vi "四段比较器（TimeStamp[]）.vi"(1 "输入时间标识":timestamp[](array[timestamp]), 2 "低":timestamp, 3 "中":timestamp, 4 "高":timestamp) -> (0 "Range":enum16{"超低", "中偏低", "中偏高", "超高"}[](array[ring]))   [LabVIEW 2011]
doc: "功能：\n\n返回一个枚举，表明输入数的范围，用于三段比较。\n\n\nCSXCS_366创建。"
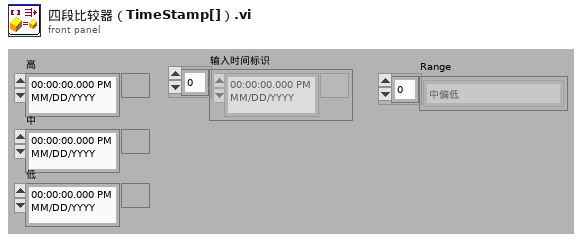
[diagram p1: front panel]
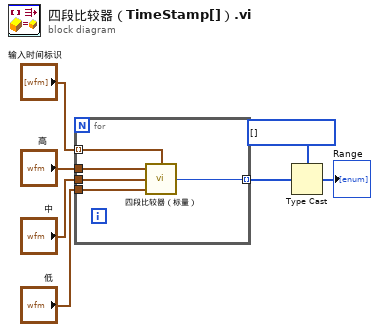
[diagram p0: block diagram]
diagram:
  w2 = enum16{"超低", "中偏低", "中偏高", "超高"}[] [] items=["超低", "中偏低", "中偏高", "超高"] ("Range")
  n1 = for {
    tunnel: "高" -> [w12]
    tunnel: "中" -> [w11]
    tunnel: "低" -> [w10]
    tunnel: "输入时间标识" -> [w9] mode=indexing
    tunnel: [w8] -> w3 mode=indexing
    n2 = call-poly "四段比较器（标量）.vi"("输入时间标识"=w9, "低"=w10, "中"=w11, "高"=w12) -> ("Range"=w8:enum16{"超低", "中偏低", "中偏高", "超高"})
  }
  n3 = Type Cast(type=w2, x=w3) -> (*(type *) &x=→"Range":enum16{"超低", "中偏低", "中偏高", "超高"}[])
